vi "题目4.vi"() -> ()   [LabVIEW 2017]
uses:
  <vilib>/measure/NI_MABase.lvlib
panel:
  out "最小值":dbl
  out "大小":i32
  out "dt":dbl
  out "Y":dbl[](array[numeric])
  out "signal out":waveform(dbl) caption="信号输出"
  in  "frequency":dbl=10.0 caption="频率" format="%.2p"
  in  "amplitude":dbl=1.0 caption="幅值" format="%.2p"
  in  "phase":dbl caption="相位" format="%.2p"
  in  "reset signal":bool caption="重置信号"
  in  "sampling info":cluster{"Fs":dbl, "#s":dbl}={"Fs"=1000.0, "#s"=1000.0} caption="采样信息" {"Fs" format="%.2p"}
  in  "offset":dbl caption="偏移量" format="%.2p"
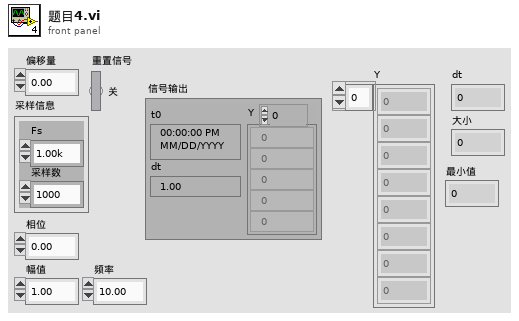
[diagram p1: front panel]
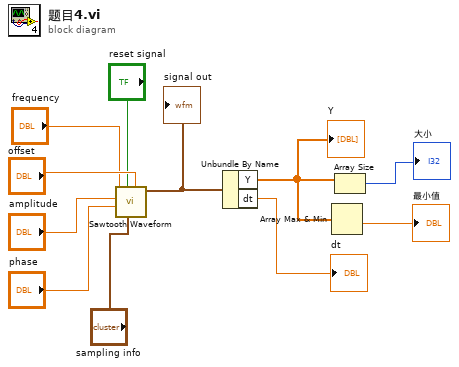
[diagram p0: block diagram]
diagram:
  n1 = call <vilib>:"Sawtooth Waveform.vi"("offset"="offset", "sampling info"="sampling info", "reset signal"="reset signal", "phase"="phase", "amplitude"="amplitude", "frequency"="frequency") -> ("signal out"=w5:waveform(dbl))  [unwired: 4 in, 1 out]
  "signal out" <- w5
  n2 = Unbundle By Name(w5) -> ("Y"=w2:dbl[], "dt"=→"dt":dbl)
  "Y" <- w2
  n3 = Array Max & Min(array=w2) -> (min value=→"最小值":dbl)  [unwired: 3 out]
  n4 = Array Size(array=w2) -> (size(s)=→"大小":i32)
